vi "FTW-Message-Lossy-Initialize.vi"(0 "FTW-Message-Lossy In":refnum<class "FTW-Message-Lossy.lvclass">, 5 "Sender Identity":string, 7 "Message Header":string, 9 "Message Body":string, 11 "error in":errorcluster) -> (4 "FTW-Message-Lossy Out":refnum<class "FTW-Message-Lossy.lvclass">, 6 "overflow?":bool, 15 "error out":errorcluster)   [LabVIEW 2013, in "FTW-Message-Lossy.lvclass"]
uses:
  FTW-Message-Lossy.lvclass
  Base/FTW-Message.lvclass
panel:
  # "Inputs"
  # "Outputs"
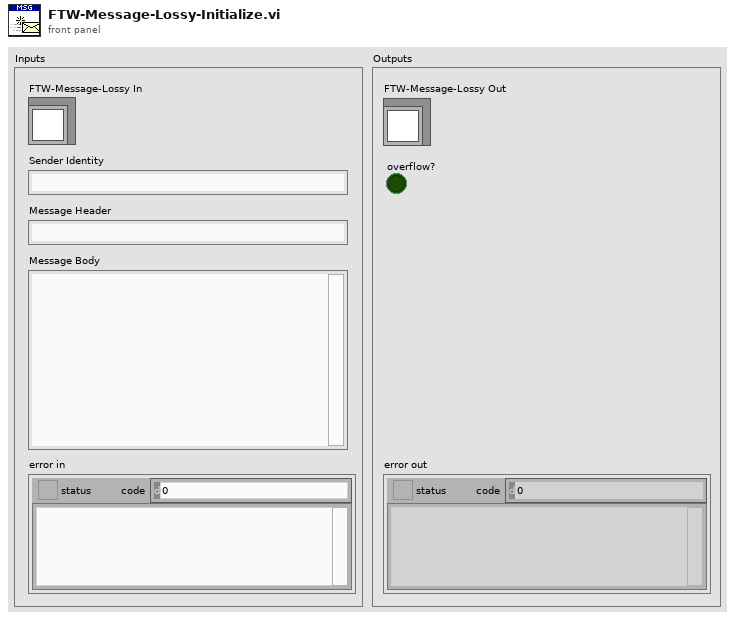
[diagram p1: front panel]
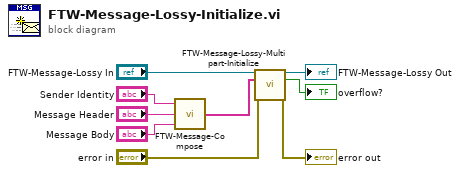
[diagram p0: block diagram]
diagram:
  n1 = call "FTW-Message-Compose.vi"("Message Body"="Message Body", "Message Header"="Message Header", "Sender Identity"="Sender Identity") -> ("Multipart Message"=w5:string[])  [unwired: 1 in]
  n2 = call-dynamic "FTW-Message-Lossy-Multipart-Initialize.vi"("FTW-Message-Lossy In"="FTW-Message-Lossy In", "Message Parts"=w5, "error in"="error in") -> ("FTW-Message-Lossy Out"=→"FTW-Message-Lossy Out":refnum<class "FTW-Message-Lossy.lvclass">, "overflow?"=→"overflow?":bool, "error out"=→"error out":errorcluster)  [unwired: 10 in]
